vi "Test Launcher DebugTerminal.vi"   [LabVIEW 2013]
uses:
  Stream Direction -- enum.ctl
  DebuggingTerminal.lvclass
types:
  T1 = typedef "MQTT Base.lvlib/DebuggingTerminal.lvclass/Stream Direction -- enum.ctl" = enum16{"Incoming", "Outgoing"}
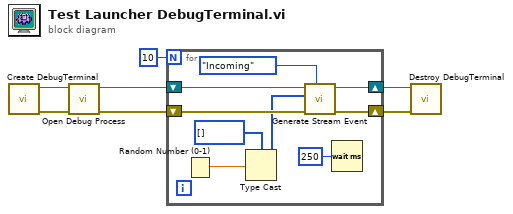
[diagram p0: block diagram]
diagram:
  n1 = call "Create DebugTerminal.vi"() -> ("error out"=w6:errorcluster, "DebuggingTerminal out"=w7:refnum<class "DebuggingTerminal.lvclass">)  [unwired: 10 in]
  n2 = call "Open Debug Process.vi"("error in (no error)"=w6, "DebuggingTerminal in"=w7) -> ("error out"=w4:errorcluster, "DebuggingTerminal out"=w5:refnum<class "DebuggingTerminal.lvclass">)  [unwired: 8 in]
  n3 = for {
    N: 10 -> [_]
    shift-right: [w13] -> w2
    shift-left: w5 -> [w16]
    shift-right: [w14] -> w3
    shift-left: w4 -> [w15]
    n4 = Random Number (0-1)() -> (number: 0 to 1=w12:dbl)
    n5 = Type Cast(type=u8[] [] ("Bytes"), x=w12) -> (*(type *) &x=w11:u8[])
    n6 = call "Generate Stream Event.vi"("Direction"=Stream_Direction_--_enum."Incoming", "error in (no error)"=w15, "Bytes"=w11, "DebuggingTerminal in"=w16) -> ("error out"=w14:errorcluster, "DebuggingTerminal out"=w13:refnum<class "DebuggingTerminal.lvclass">)  [unwired: 6 in]
    n7 = Wait (ms)(milliseconds to wait=u32 250) -> ()  [unwired: 1 out]
  }
  n8 = call "Destroy DebugTerminal.vi"("error in (no error)"=w3, "DebuggingTerminal in"=w2) -> ()  [unwired: 8 in, 2 out]
